vi "StageReady.vi"(8 "error in (no error)":errorcluster, 11 "Microscope in":refnum<class "Microscope.lvclass">) -> (0 "error out":errorcluster, 3 "Microscope out":refnum<class "Microscope.lvclass">)   [LabVIEW 2012, in "Microscope.lvclass"]
uses:
  classes/Microscope.lvclass
  typedefs/Move Type.ctl
  classes/Microscope.lvclass/Microscope.ctl
  variables/GlobalUI.vi
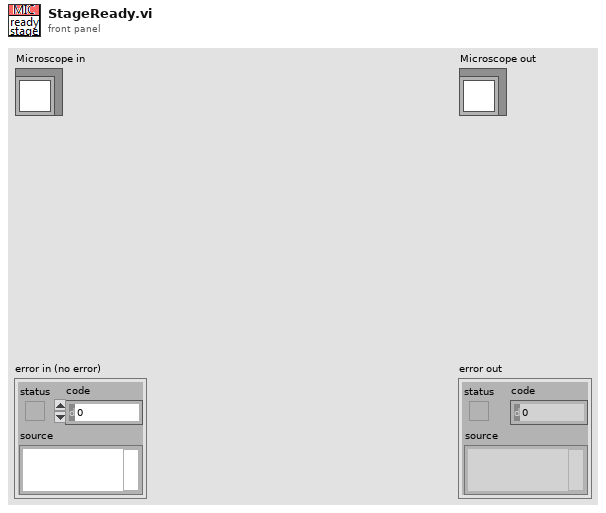
[diagram p1: front panel]
types:
  T1 = typedef "Move Type.ctl" = enum16{"None", "Continuous", "Discrete"}
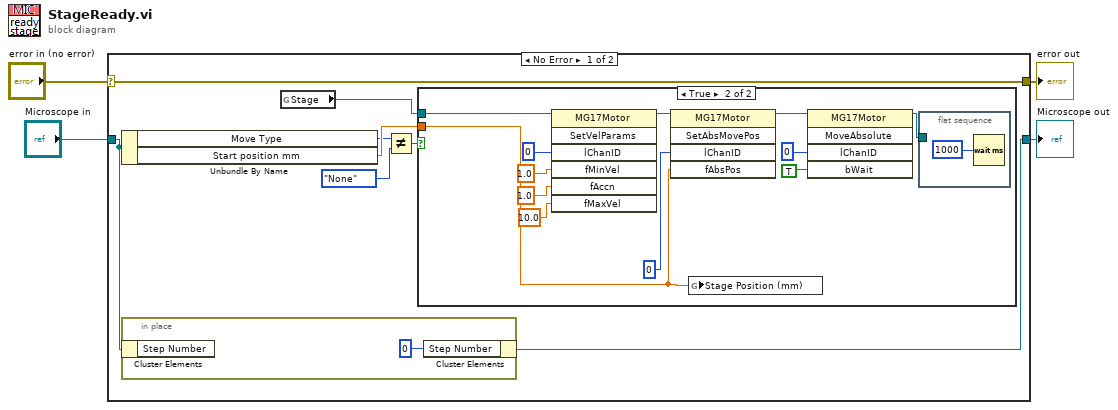
[diagram p0: block diagram]
diagram:
  n1 = case shown="No Error" "error in (no error)" {
    selector: "error in (no error)" -> [w11 w28]
    tunnel: [w11 w28] -> w3
    tunnel: [w9 w27] -> w1
    tunnel: "Microscope in" -> [w10 w27]
    frame No Error {
      n2 = Unbundle By Name(w10) -> ("Move Type"=w8:T1, "Start position mm"=w12:dbl)
      n3 = in-place {
        n4 = in-place-cluster #1(w10) -> ()  [unwired: 1 out]
        n5 = in-place-cluster #1("Step Number"=0) -> (w9:refnum<class "Microscope.lvclass">)
      }
      n6 = global read "GlobalUI.vi" "Stage"() -> (w5:refnum<k7>)
      n7 = Not Equal?(x=w8, y=Move_Type."None") -> (x != y?=w6:bool)
      n8 = case shown="True" w6 {
        tunnel: w12 -> [_ w14]
        tunnel: w5 -> [_ w20]
        frame False {
        }
        frame True {
          n9 = invoke class="MG17Motor" method="SetVelParams"(reference=w20, "lChanID"=0, "fMinVel"=sgl 1.0, "fAccn"=sgl 1.0, "fMaxVel"=sgl 10.0) -> (reference out=w21:refnum<k7>)  [unwired: 2 in, 6 out]
          n10 = invoke class="MG17Motor" method="SetAbsMovePos"(reference=w21, "lChanID"=0, "fAbsPos"=w14) -> (reference out=w22:refnum<k7>)  [unwired: 2 in, 4 out]
          n11 = global write "GlobalUI.vi" "Stage Position (mm)"(w14) -> ()
          n12 = invoke class="MG17Motor" method="MoveAbsolute"(reference=w22, "lChanID"=0, "bWait"=TRUE) -> (reference out=w15:refnum<k7>)  [unwired: 2 in, 4 out]
          n13 = flat-sequence {
            tunnel: w15 -> [_]
            frame #0 {
              n14 = Wait (ms)(milliseconds to wait=u32 1000) -> ()  [unwired: 1 out]
            }
          }
        }
      }
    }
    frame Error {
    }
  }
  "error out" <- w3
  "Microscope out" <- w1
